vi "Open Object.vi"(8 "Error In":errorcluster, 9 "queue IN":refnum<queue>, 10 "Tree Path":string[](array[string]), 11 "WAD Cluster IN":T1) -> (0 "Error Out":errorcluster, 1 "queue OUT":refnum<queue>, 3 "WAD Cluster OUT":T1)   [LabVIEW 2017]
uses:
  WAD_MainCluster.ctl
  TextureList.ctl
  PatchList.ctl
  Lumps.ctl
  <vilib>/picture/picture.llb/Draw 8-Bit Pixmap.vi
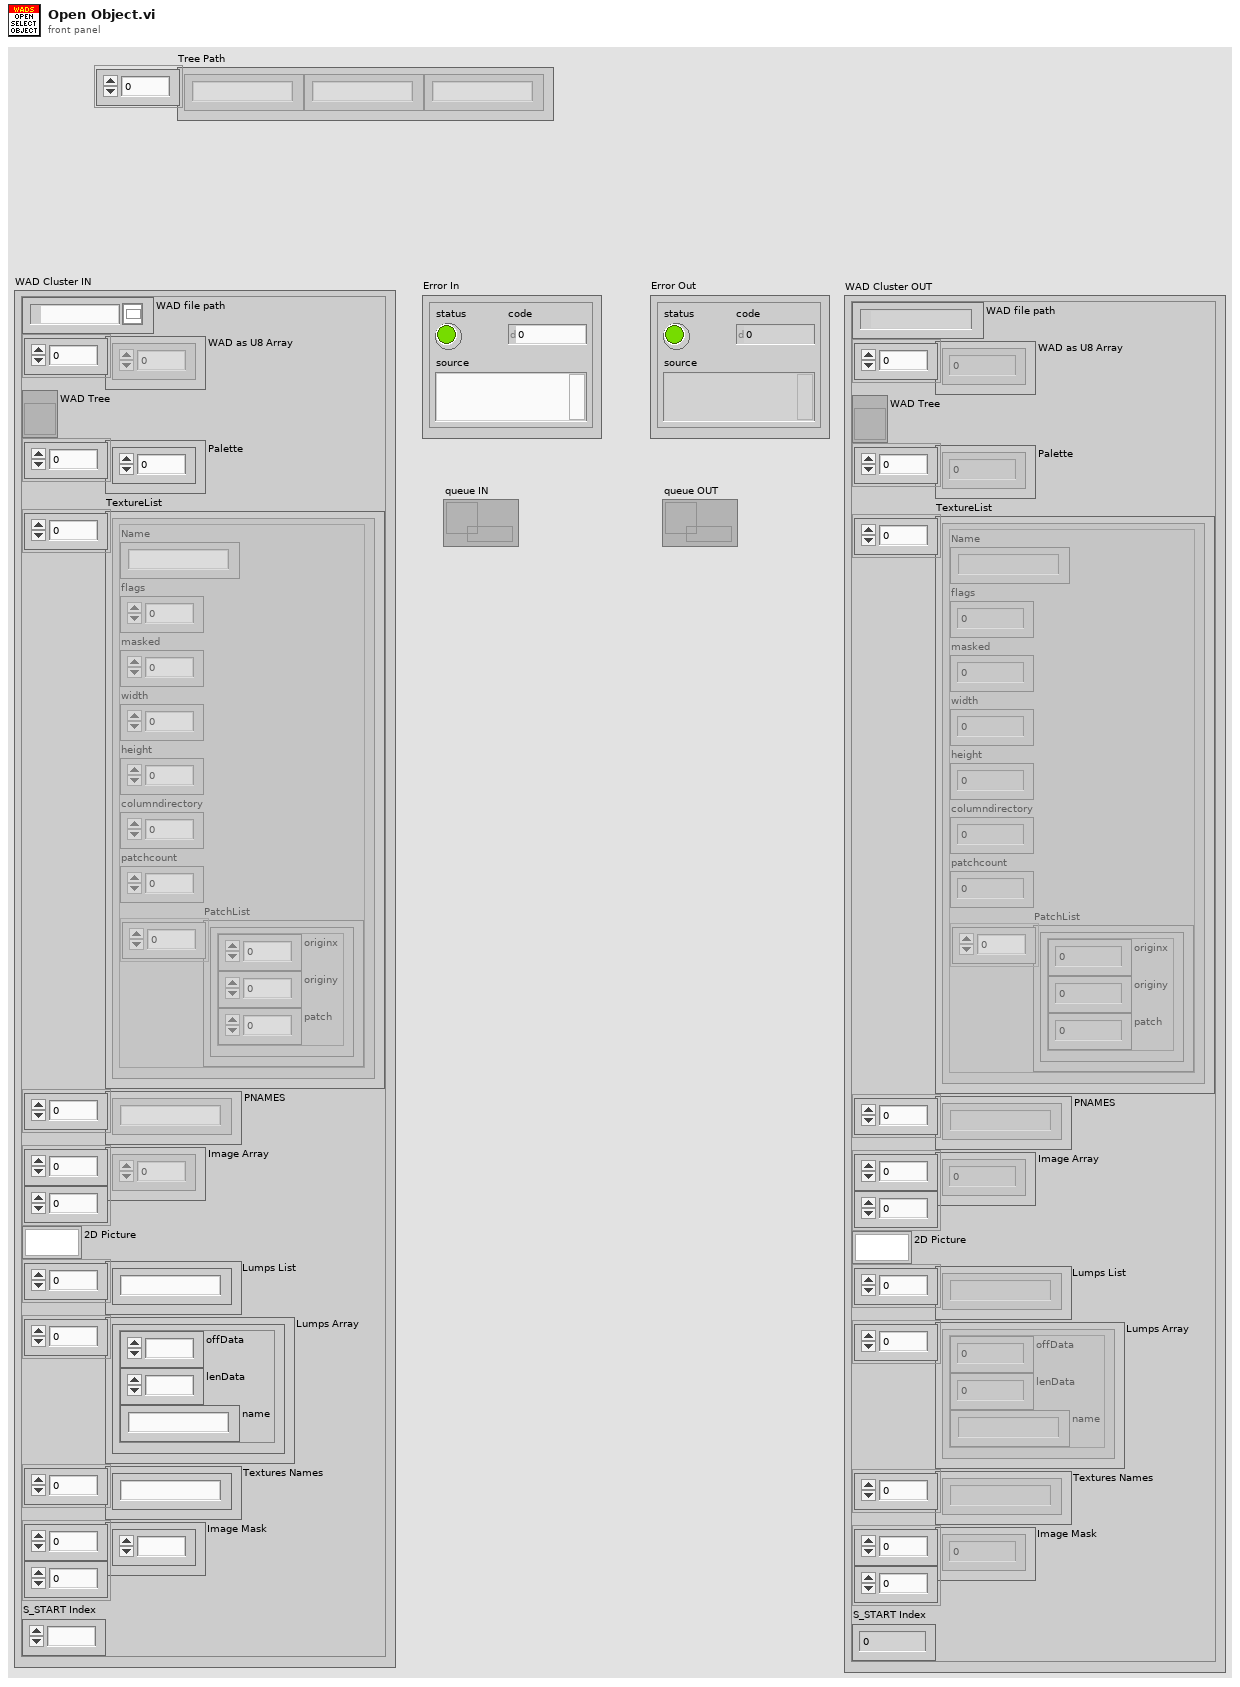
[diagram p1: front panel]
types:
  T1 = typedef "WAD_MainCluster.ctl" = cluster{"WAD file path":path, "WAD as U8 Array":u8[], "WAD Tree":refnum<vi>, "Palette":u32[], "TextureList":T2[], "PNAMES":string[], "Image Array":i16[][], "2D Picture":picture, "Lumps List":string[], "Lumps Array":T4[], "Textures Names":string[], "Image Mask":i16[][], "S_START Index":i32}
  T2 = typedef "TextureList.ctl" = cluster{"Name":string, "flags":u16, "masked":i16, "width":i16, "height":i16, "columndirectory":u32, "patchcount":i16, "PatchList":T3[]}
  T3 = typedef "PatchList.ctl" = cluster{"originx":i16, "originy":i16, "patch":i16}
  T4 = typedef "Lumps.ctl" = cluster{"offData":i32, "lenData":i32, "name":string}
  T5 = cluster{"Font Name:":string, "Size":i16, "Strikeout?":bool, "Italic?":bool, "Underline?":bool, "Outline?":bool, "Shadow?":bool, "Bold?":bool}
  T6 = typedef "PatchHeader.ctl" = cluster{"Width":u16, "Height":u16, "XOffset":i16, "YOffset":i16}
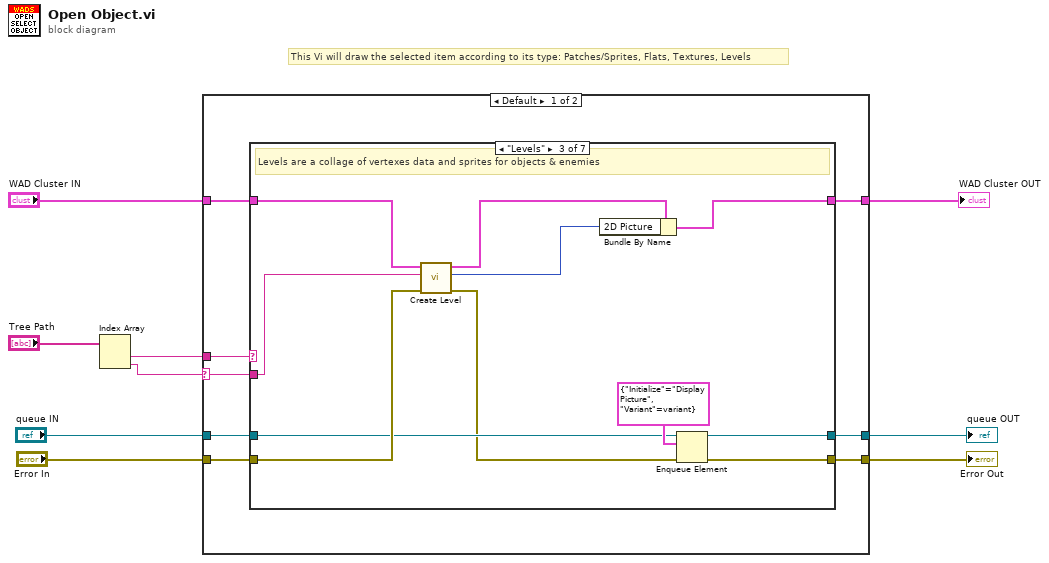
[diagram p0: block diagram]
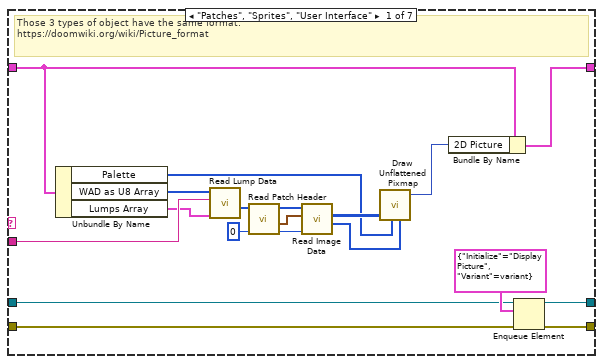
[diagram p2: hidden frame]
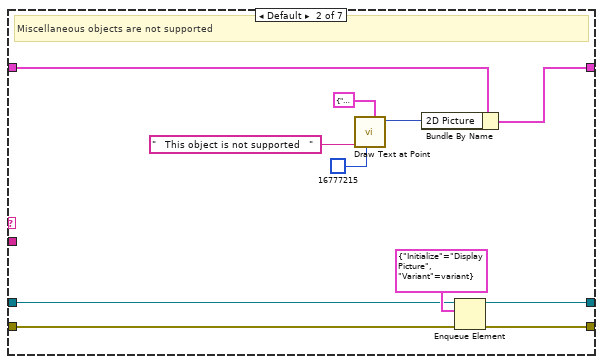
[diagram p3: hidden frame]
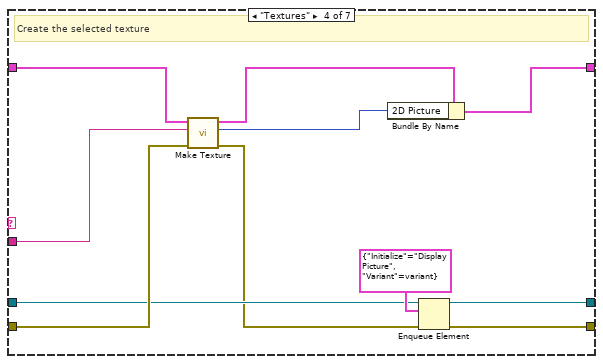
[diagram p4: hidden frame]
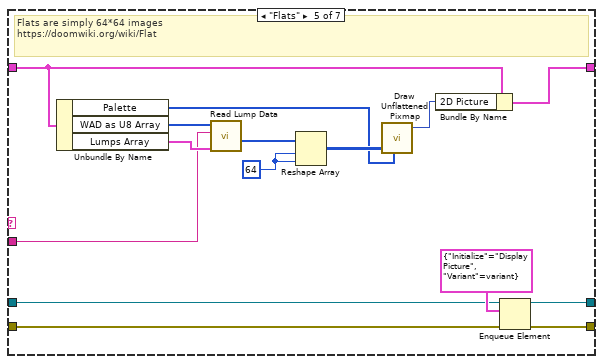
[diagram p5: hidden frame]
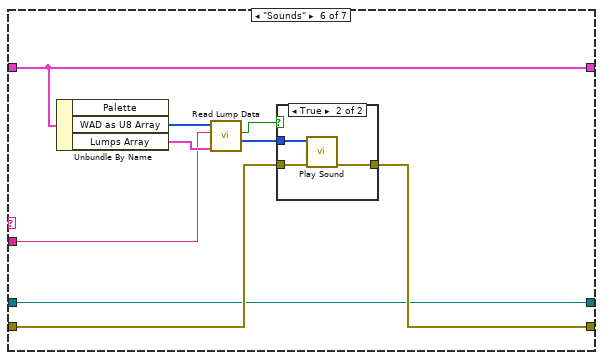
[diagram p6: hidden frame]
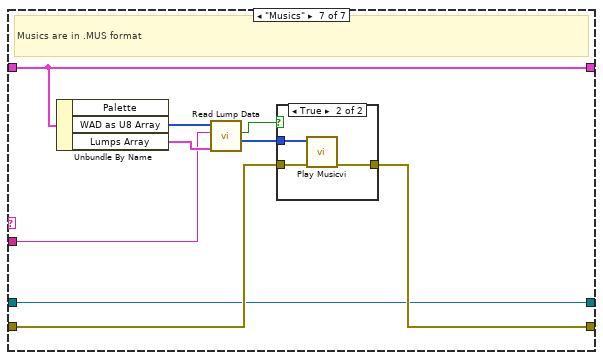
[diagram p8: hidden frame]
diagram:
  # "This Vi will draw the selected item according to its type: Patches/Sprites, Flats, Textures, Levels"
  n1 = Index Array(array="Tree Path") -> (element #1=w8:string, element #2=w3:string)  [unwired: 2 in]
  n2 = case shown="Default" w3 {
    selector: w3 -> [w12 _]
    tunnel: w8 -> [w17 _]
    tunnel: "WAD Cluster IN" -> [w16 w113]
    tunnel: [w15 w113] -> w6
    tunnel: "Error In" -> [w14 w112]
    tunnel: [w13 w112] -> w4
    tunnel: [w11 w111] -> w2
    tunnel: "queue IN" -> [w10 w111]
    frame Default {
      n3 = case shown="\"Levels\"" w17 {
        tunnel: w16 -> [w25 w44 w58 w69 w77 w90 w103]
        tunnel: [w23 w42 w53 w64 w75 w90 w103] -> w15
        tunnel: w14 -> [w20 w39 w57 w67 w72 w87 w100]
        tunnel: [w19 w37 w49 w60 w70 w86 w99] -> w13
        tunnel: w12 -> [w35 _ w56 w68 w82 w91 w104]
        tunnel: [w18 w38 w48 w59 w71 w85 w98] -> w11
        tunnel: w10 -> [w21 w40 w51 w62 w73 w85 w98]
        frame "Patches", "Sprites", "User Interface" {
          # "Those 3 types of object have the same format:\nhttps://doomwiki.org/wiki/Picture_format"
          n4 = Unbundle By Name(w25) -> ("Palette"=w26:u32[], "WAD as U8 Array"=w36:u8[], "Lumps Array"=w34:T4[])
          n5 = call "Read Lump Data.vi"("Lumps Directory IN"=w34, "Lump Name"=w35, "Input U8"=w36) -> ("Lump DATA OUT"=w33:u8[])  [unwired: 5 in, 3 out]
          n6 = call "Read Patch Header.vi"("Index"=u32 0, "Patch DATA IN"=w33) -> ("Index+8"=w31:u32, "PatchHeader"=w30:T6, "Patch DATA OUT"=w32:u8[])  [unwired: 7 in]
          n7 = call "Read Image Data.vi"("Input Index"=w31, "PatchHeader"=w30, "Patch DATA IN"=w32) -> ("Mask OUT"=w27:u8[], "Image OUT"=w28:u8[][])  [unwired: 5 in, 2 out]
          n8 = call-poly <vilib>:"Draw Unflattened Pixmap.vi"("data"=w28, "color table"=w26, "mask"=w27) -> ("new picture"=w24:picture)  [unwired: 6 in]
          n9 = Bundle By Name(cluster=w25, "2D Picture"=w24) -> (w23:T1)
          n10 = Enqueue Element(queue=w21, element=cluster{"Initialize":string, "Variant":variant} {"Initialize"="Display Picture", "Variant"=variant}, error in (no error)=w20) -> (queue out=w18:refnum<queue>, error out=w19:errorcluster)  [unwired: 1 in, 1 out]
        }
        frame Default {
          # "Miscellaneous objects are not supported"
          n11 = call <vilib>:"Draw Text at Point.vi"("[user-specified font]"=T5 {"Font Name:"="", "Size"=12, "Strikeout?"=FALSE, "Italic?"=FALSE, "Underline?"=FALSE, "Outline?"=FALSE, "Shadow?"=TRUE, "Bold?"=TRUE}, "text color(black)"=u32 16777215, "text"="   This object is not supported   " ("String")) -> ("new picture"=w43:picture)  [unwired: 7 in, 1 out]
          n12 = Bundle By Name(cluster=w44, "2D Picture"=w43) -> (w42:T1)
          n13 = Enqueue Element(queue=w40, element=cluster{"Initialize":string, "Variant":variant} {"Initialize"="Display Picture", "Variant"=variant}, error in (no error)=w39) -> (queue out=w38:refnum<queue>, error out=w37:errorcluster)  [unwired: 1 in, 1 out]
        }
        frame "Levels" {
          # "Levels are a collage of vertexes data and sprites for objects & enemies"
          n14 = call "Create Level.vi"("Error In"=w57, "Selected Level"=w56, "WAD Cluster IN"=w58) -> ("Error Out"=w50:errorcluster, "2D Picture"=w54:picture, "WAD Cluster OUT"=w55:T1)  [unwired: 6 in]
          n15 = Bundle By Name(cluster=w55, "2D Picture"=w54) -> (w53:T1)
          n16 = Enqueue Element(queue=w51, element=cluster{"Initialize":string, "Variant":variant} {"Initialize"="Display Picture", "Variant"=variant}, error in (no error)=w50) -> (queue out=w48:refnum<queue>, error out=w49:errorcluster)  [unwired: 1 in, 1 out]
        }
        frame "Textures" {
          # "Create the selected texture"
          n17 = call "Make Texture.vi"("Error In"=w67, "Texture Name"=w68, "WAD Cluster IN"=w69) -> ("Error Out"=w61:errorcluster, "2D Picture"=w65:picture, "WAD Cluster OUT"=w66:T1)  [unwired: 6 in]
          n18 = Bundle By Name(cluster=w66, "2D Picture"=w65) -> (w64:T1)
          n19 = Enqueue Element(queue=w62, element=cluster{"Initialize":string, "Variant":variant} {"Initialize"="Display Picture", "Variant"=variant}, error in (no error)=w61) -> (queue out=w59:refnum<queue>, error out=w60:errorcluster)  [unwired: 1 in, 1 out]
        }
        frame "Flats" {
          w80 = 64
          # "Flats are simply 64*64 images\nhttps://doomwiki.org/wiki/Flat"
          n20 = Unbundle By Name(w77) -> ("Palette"=w78:u32[], "WAD as U8 Array"=w84:u8[], "Lumps Array"=w83:T4[])
          n21 = call "Read Lump Data.vi"("Lumps Directory IN"=w83, "Lump Name"=w82, "Input U8"=w84) -> ("Lump DATA OUT"=w81:u8[])  [unwired: 5 in, 3 out]
          n22 = Reshape Array(w81, w80, w80) -> (w79:u8[][])
          n23 = call-poly <vilib>:"Draw Unflattened Pixmap.vi"("data"=w79, "color table"=w78) -> ("new picture"=w76:picture)  [unwired: 7 in]
          n24 = Bundle By Name(cluster=w77, "2D Picture"=w76) -> (w75:T1)
          n25 = Enqueue Element(queue=w73, element=cluster{"Initialize":string, "Variant":variant} {"Initialize"="Display Picture", "Variant"=variant}, error in (no error)=w72) -> (queue out=w71:refnum<queue>, error out=w70:errorcluster)  [unwired: 1 in, 1 out]
        }
        frame "Sounds" {
          n26 = Unbundle By Name(w90) -> ("WAD as U8 Array"=w93:u8[], "Lumps Array"=w92:T4[])  [unwired: 1 out]
          n27 = call "Read Lump Data.vi"("Lumps Directory IN"=w92, "Lump Name"=w91, "Input U8"=w93) -> ("Lump DATA OUT"=w89:u8[], "Found?"=w88:bool)  [unwired: 5 in, 2 out]
          n28 = case shown="True" w88 {
            tunnel: w89 -> [_ w97]
            tunnel: w87 -> [w94 w96]
            tunnel: [w94 w95] -> w86
            frame False {
            }
            frame True {
              n29 = call "Play Sound.vi"("error in (no error)"=w96, "Sound LUMP IN"=w97) -> ("error out"=w95:errorcluster)  [unwired: 9 in]
            }
          }
        }
        frame "Musics" {
          # "Musics are in .MUS format"
          n30 = Unbundle By Name(w103) -> ("WAD as U8 Array"=w106:u8[], "Lumps Array"=w105:T4[])  [unwired: 1 out]
          n31 = call "Read Lump Data.vi"("Lumps Directory IN"=w105, "Lump Name"=w104, "Input U8"=w106) -> ("Lump DATA OUT"=w102:u8[], "Found?"=w101:bool)  [unwired: 5 in, 2 out]
          n32 = case shown="True" w101 {
            tunnel: w102 -> [_ w110]
            tunnel: w100 -> [w107 w109]
            tunnel: [w107 w108] -> w99
            frame False {
            }
            frame True {
              n33 = call "Play Musicvi.vi"("error in (no error)"=w109, "Sound LUMP IN"=w110) -> ("error out"=w108:errorcluster)  [unwired: 9 in]
            }
          }
        }
      }
    }
    frame "" {
    }
  }
  "WAD Cluster OUT" <- w6
  "Error Out" <- w4
  "queue OUT" <- w2
